vi "Setting.vi"(8 "error in (no error)":errorcluster) -> (0 "error out":errorcluster)   [LabVIEW 2017]
uses:
  <vilib>/Utility/miscctls.llb/LVRowAndColumnTypeDef.ctl
  <vilib>/Utility/miscctls.llb/LVBoundsTypeDef.ctl
  <vilib>/addons/database/Connection.llb/DB Tools Open Connec (Path).vi
  <vilib>/addons/database/NI_Database_API.lvlib
panel:
  in  "Back 2":bool
  out "subarray":string[](array[string])
  in  "Select Function":string(combo)
  in  "Select Station":string(combo)
  in  "Enter CID":string
  out "Table":string[][](table)
  in  "Add CID":bool
  # "CID To ASSIGN STATIONS"
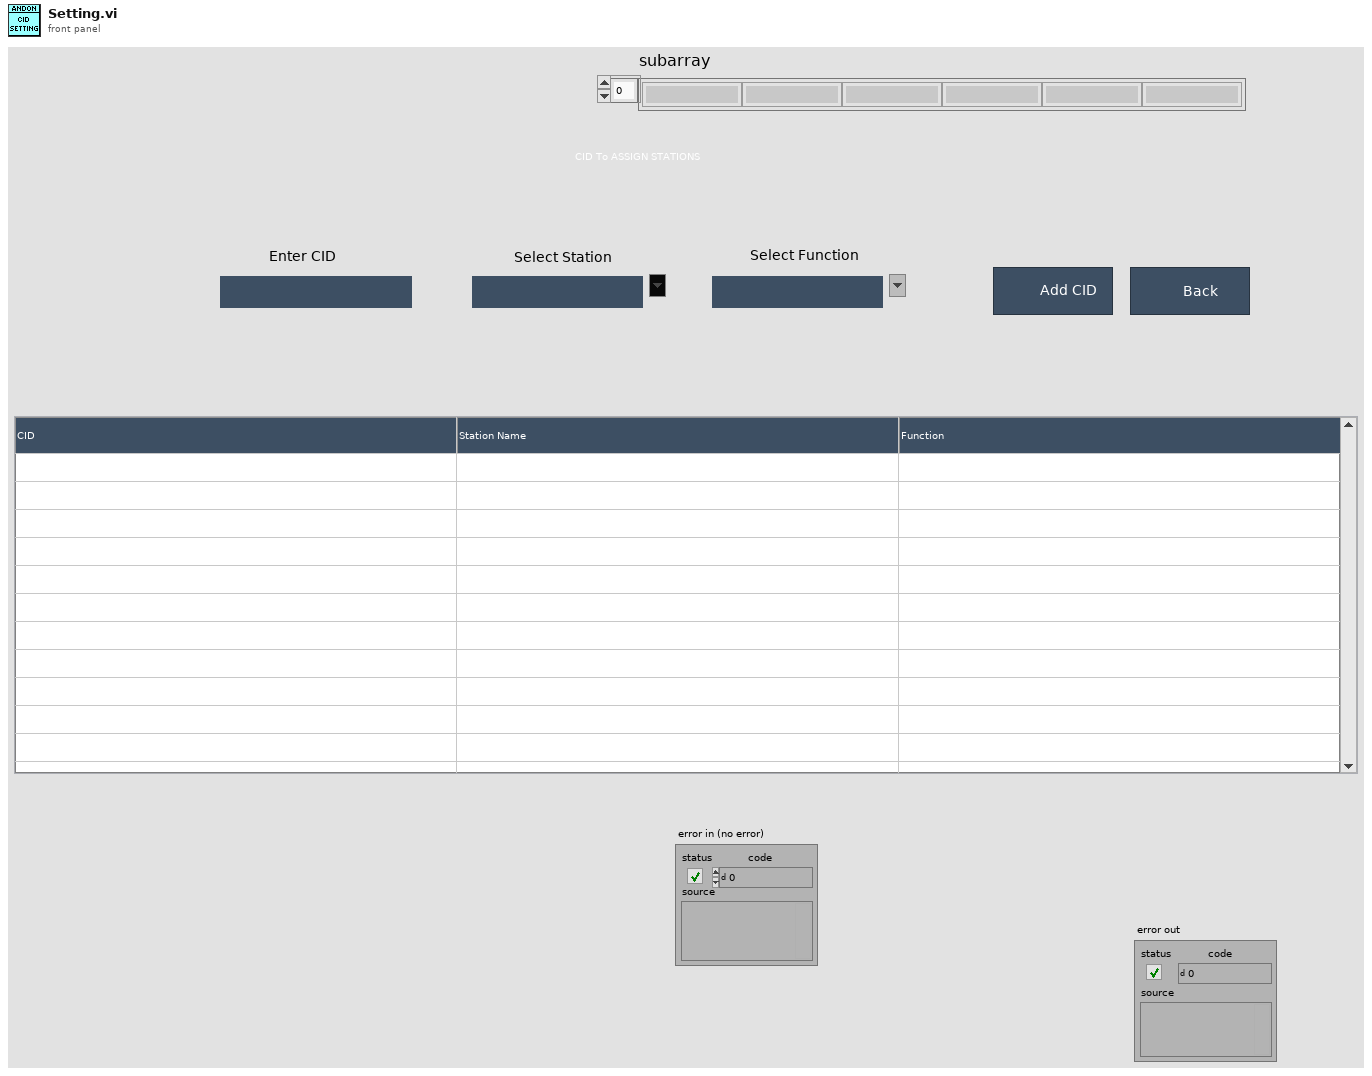
[diagram p1: front panel]
types:
  T1 = typedef "LVBoundsTypeDef.ctl" = cluster{"Width":u32, "Height":u32}
  T2 = typedef "LVRowAndColumnTypeDef.ctl" = cluster{"Row":i32, "Column":i32}
  T3 = typedef "NI_Database_API.lvlib/Conn ObjectReference.ctl" = refnum<k1>
  T4 = cluster{"Enter CID":string, i32, "Select Function ":string}
  T5 = enum32{"invalid app kind", "Development System", "Run Time System", "Student Edition", "Embedded LabVIEW", "Evaluation", "Custom"}
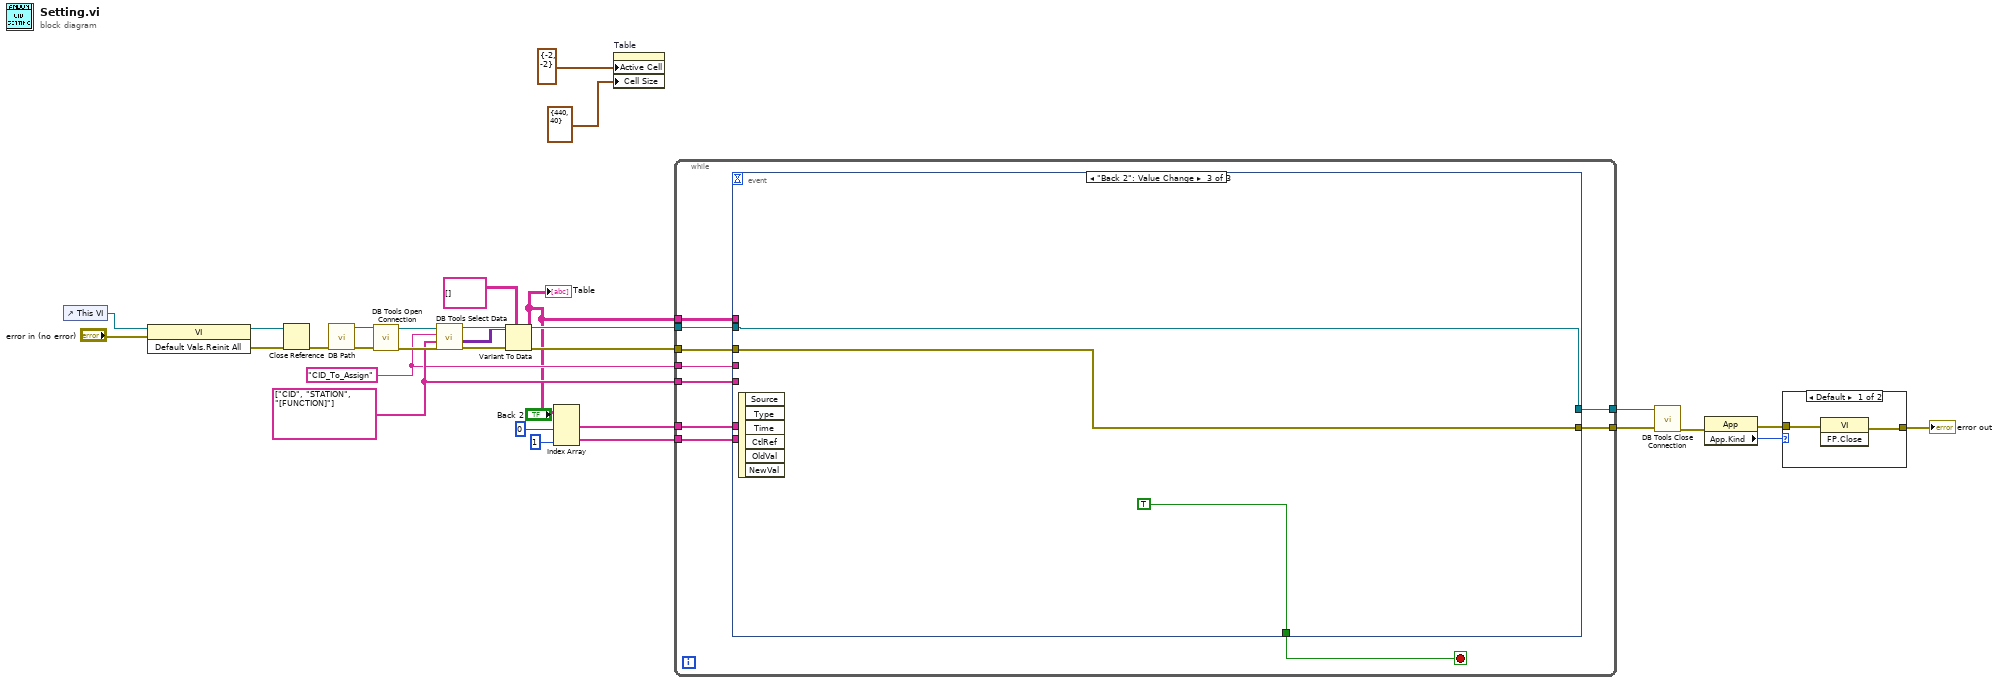
[diagram p0: block diagram]
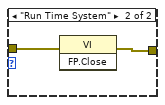
[diagram p2: hidden frame]
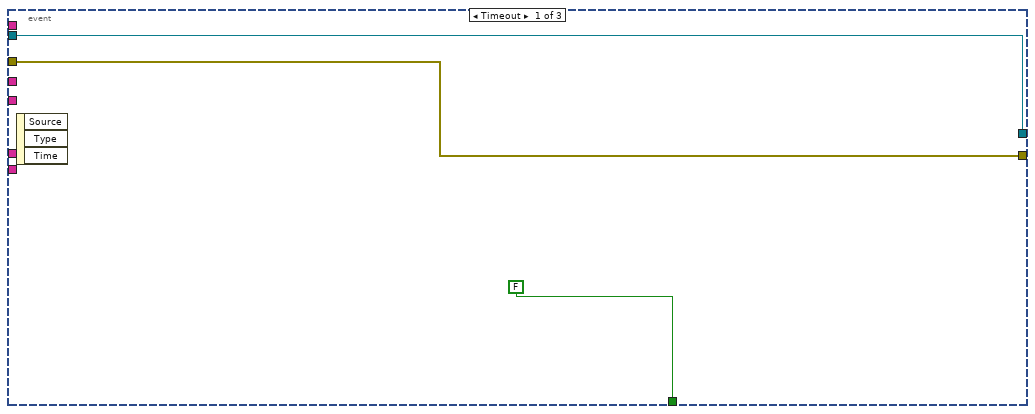
[diagram p3: hidden frame]
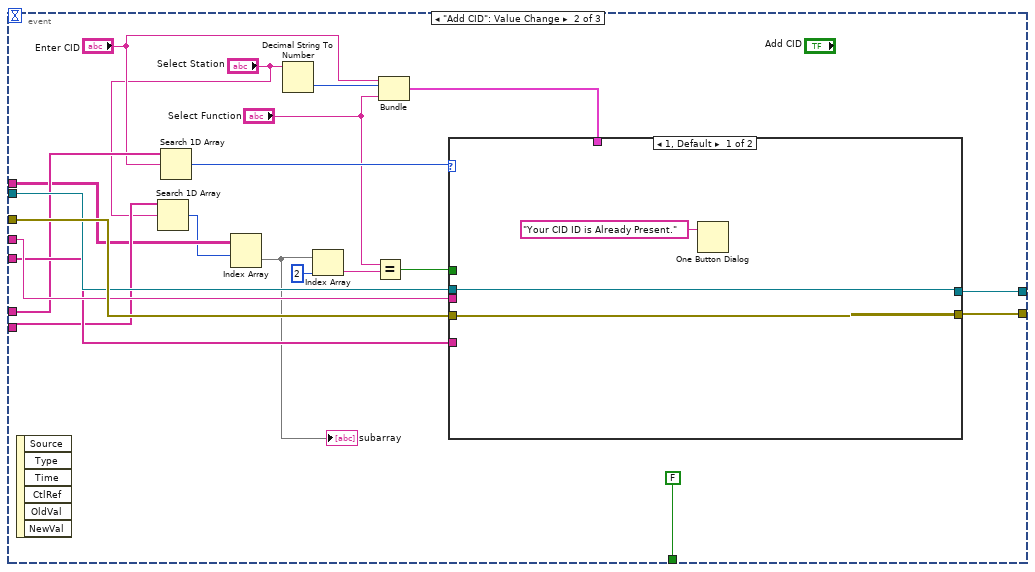
[diagram p4: hidden frame]
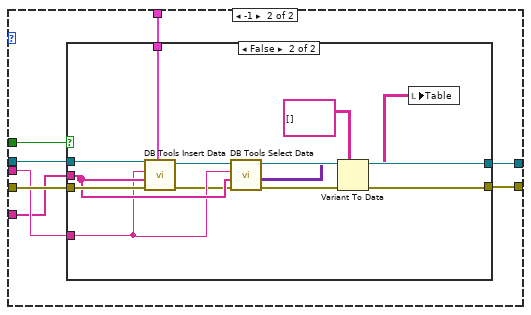
[diagram p5: hidden frame]
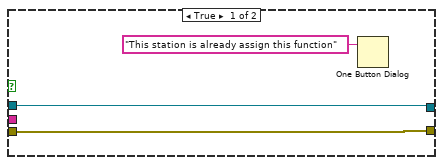
[diagram p6: hidden frame]
diagram:
  w14 = string[] ["CID", "STATION", "[FUNCTION]"] ("columns")
  w13 = "CID_To_Assign" ("table")
  n1 = control-ref of="This VI"() -> (w27:refnum<vi>)
  n2 = invoke class="VI" method="Default Vals.Reinit All"(reference=w27, error in="error in (no error)") -> (reference out=w24:refnum<vi>, error out=w25:errorcluster)  [unwired: 1 in, 1 out]
  n3 = Close Reference(reference=w24, error in (no error)=w25) -> (error out=w20:errorcluster)
  n4 = call "DB Path.vi"("error in"=w20) -> ("error out"=w19:errorcluster, "DB Path"=w18:path)  [unwired: 9 in]
  n5 = call-poly <vilib>:"DB Tools Open Connection.vi"("error in (no error)"=w19, "connection information"=w18) -> ("error out"=w17:errorcluster, "connection reference"=w16:T3)  [unwired: 6 in]
  n6 = call <vilib>:"DB Tools Select Data.vi"("error in (no error)"=w17, "columns"=w14, "table"=w13, "connection reference"=w16) -> ("error out"=w12:errorcluster, "data"=w10:variant[][], "connection reference out"=w15:T3)  [unwired: 2 in]
  n7 = Variant To Data(error in=w12, type=string[][] [], Variant=w10) -> (data=w4:string[][], error out=w11:errorcluster)
  "Table" <- w4
  n8 = Index Array(array=w4, index (col) #1=0 ("disabled index (col)"), index (col) #2=1 ("index (col)")) -> (element #1=w7:string[], element #2=w5:string[])  [unwired: 2 in]
  n9 = property on="Table" class="Tbl (strict)"("Active Cell"=T2 {"Row"=-2, "Column"=-2} ("Active Cell:Active Cell"), "Cell Size"=T1 {"Width"=440, "Height"=40} ("Active Cell:Cell Size")) -> ()  [unwired: 2 in, 2 out]
  n10 = while {
    tunnel: w11 -> [w39]
    tunnel: w15 -> [w38]
    tunnel: [w37] -> w2
    tunnel: [w36] -> w3
    tunnel: w14 -> [w35]
    tunnel: w13 -> [w34]
    tunnel: w7 -> [w32]
    tunnel: w5 -> [w31]
    tunnel: w4 -> [w30]
    stop <- w33 stop-if-true
    n11 = event shown="[2] \"Back 2\": Value Change" {
      selector: _ -> [_ _ _]
      dyn-events: _ -> [_ _ _]
      timeout: _ -> [_ _ _]
      tunnel: w39 -> [w41 w63 w92]
      tunnel: w38 -> [w40 w62 w93]
      tunnel: [w41 w58 w92] -> w37
      tunnel: [w40 w61 w93] -> w36
      tunnel: w35 -> [_ w59 _]
      tunnel: w34 -> [_ w60 _]
      tunnel: [FALSE FALSE TRUE] -> w33
      tunnel: w32 -> [_ w57 _]
      tunnel: w31 -> [_ w52 _]
      tunnel: w30 -> [_ w49 _]
      event Timeout {
        n12 = event-data() -> ()  [unwired: 1 in, 3 out]
      }
      event "Add CID": Value Change {
        n13 = event-data() -> ()  [unwired: 1 in, 6 out]
        n14 = Search 1D Array(1D array=w52, element="Select Station") -> (index of element=w43:i32)  [unwired: 1 in]
        n15 = Search 1D Array(1D array=w57, element="Enter CID") -> (index of element=w55:i32)  [unwired: 1 in]
        n16 = Index Array(array=w49, index (row)=w43) -> (element=w44:string[])  [unwired: 1 in]
        "subarray" <- w44
        n17 = Decimal String To Number(string="Select Station") -> (number=w53:i32)  [unwired: 2 in, 1 out]
        n18 = Index Array(array=w44, index=2) -> (element=w46:string)
        n19 = Equal?(x="Select Function", y=w46) -> (x = y?=w47:bool)
        n20 = Bundle("Enter CID"="Enter CID", w53, "Select Function"="Select Function") -> (w56:T4)  [unwired: 1 in]
        n21 = case shown="1, Default" w55 {
          tunnel: w63 -> [w66 w74]
          tunnel: w62 -> [w65 w73]
          tunnel: [w65 w72] -> w61
          tunnel: w60 -> [_ w71]
          tunnel: w59 -> [_ w70]
          tunnel: [w66 w69] -> w58
          tunnel: w56 -> [_ w68]
          tunnel: w47 -> [_ w67]
          frame 1, Default {
            n22 = One Button Dialog(message="Your CID ID is Already Present.") -> ()  [unwired: 1 in, 1 out]
          }
          frame -1 {
            n23 = case shown="False" w67 {
              tunnel: w74 -> [w77 w90]
              tunnel: w73 -> [w76 w89]
              tunnel: [w76 w88] -> w72
              tunnel: w71 -> [_ w84]
              tunnel: w70 -> [_ w87]
              tunnel: [w77 w86] -> w69
              tunnel: w68 -> [_ w85]
              frame True {
                n24 = One Button Dialog(message="This station is already assign this function") -> ()  [unwired: 1 in, 1 out]
              }
              frame False {
                n25 = call <vilib>:"DB Tools Insert Data.vi"("data"=w85, "error in (no error)"=w90, "columns"=w87, "table"=w84, "connection reference"=w89) -> ("error out"=w82:errorcluster, "connection reference out"=w83:T3)  [unwired: 5 in]
                n26 = call <vilib>:"DB Tools Select Data.vi"("error in (no error)"=w82, "columns"=w87, "table"=w84, "connection reference"=w83) -> ("error out"=w81:errorcluster, "data"=w79:variant[][], "connection reference out"=w88:T3)  [unwired: 2 in]
                n27 = Variant To Data(error in=w81, type=string[][] [], Variant=w79) -> (data=w78:string[][], error out=w86:errorcluster)
                n28 = local write "Table"(w78) -> ()
              }
            }
          }
        }
      }
      event "Back 2": Value Change {
        n29 = event-data() -> ()  [unwired: 1 in, 6 out]
      }
    }
  }
  n30 = call <vilib>:"DB Tools Close Connection.vi"("error in (no error)"=w2, "connection reference"=w3) -> ("error out"=w1:errorcluster)  [unwired: 5 in]
  n31 = property class="App"(error in=w1) -> (error out=w22:errorcluster, "App.Kind"=w23:T5)  [unwired: 1 in, 1 out]
  n32 = case shown="Default" w23 {
    tunnel: w22 -> [w95 w97]
    tunnel: [w94 w96] -> w21
    frame Default {
      n33 = invoke class="VI" method="FP.Close"(error in=w95) -> (error out=w94:errorcluster)  [unwired: 2 in, 2 out]
    }
    frame "Run Time System" {
      n34 = invoke class="VI" method="FP.Close"(error in=w97) -> (error out=w96:errorcluster)  [unwired: 2 in, 2 out]
    }
  }
  "error out" <- w21
